vi "SubVI_Overlay Result.vi"(8 "Error in":errorcluster, 9 "Parameter_String":T1={"Font, Size & Style"={"Desired Font (Application)"=enum."Application Font", "[User-specified Font]"={"Font Name"="", "Size"=12, "Strikeout?"=FALSE, "Italic?"=FALSE, "Underline?"=FALSE, "Outline?"=FALSE, "Shadow?"=FALSE, "Bold?"=FALSE, "Rotation Angle"=0.0}, "Horizontal Alignment"=0, "Vertical Alignment"=0}, "Position"={"Image X %"=5.0, "Image Y %"=5.0}} {"Position"."Image Y %" min=5 max=95 step=5; "Position"."Image X %" min=5 max=95 step=5; "Font, Size & Style"."Vertical Alignment" items=["Bottom", "Top", "Baseline"]; "Font, Size & Style"."Horizontal Alignment" items=["Left", "Center", "Right"]; "Font, Size & Style"."[User-specified Font]"."Rotation Angle" format="%.2f"}, 10 "Result Array":T3(array[cluster]), 11 "Image In":T2) -> ()   [LabVIEW 2013]
uses:
  <vilib>/vision/Image Controls.llb/IMAQ Image.ctl
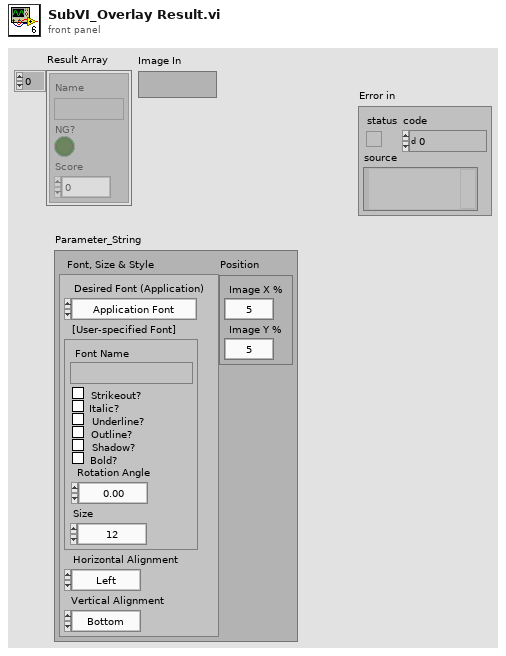
[diagram p1: front panel]
types:
  T1 = cluster{"Font, Size & Style":cluster{"Desired Font (Application)":enum16{"User-specified Font", "Application Font", "System Font", "Dialog Font"}, "[User-specified Font]":cluster{"Font Name":string, "Size":i16, "Strikeout?":bool, "Italic?":bool, "Underline?":bool, "Outline?":bool, "Shadow?":bool, "Bold?":bool, "Rotation Angle":dbl}, "Horizontal Alignment":i16, "Vertical Alignment":i16}, "Position":cluster{"Image X %":sgl, "Image Y %":sgl}}
  T2 = typedef "IMAQ Image.ctl" = refnum<image>
  T3 = cluster{"Name":string, "NG?":bool, "Score":dbl}[]
  T4 = cluster{"Desired Font (Application)":enum16{"User-specified Font", "Application Font", "System Font", "Dialog Font"}, "[User-specified Font]":cluster{"Font Name":string, "Size":i16, "Strikeout?":bool, "Italic?":bool, "Underline?":bool, "Outline?":bool, "Shadow?":bool, "Bold?":bool, "Rotation Angle":dbl}, "Horizontal Alignment":i16, "Vertical Alignment":i16}
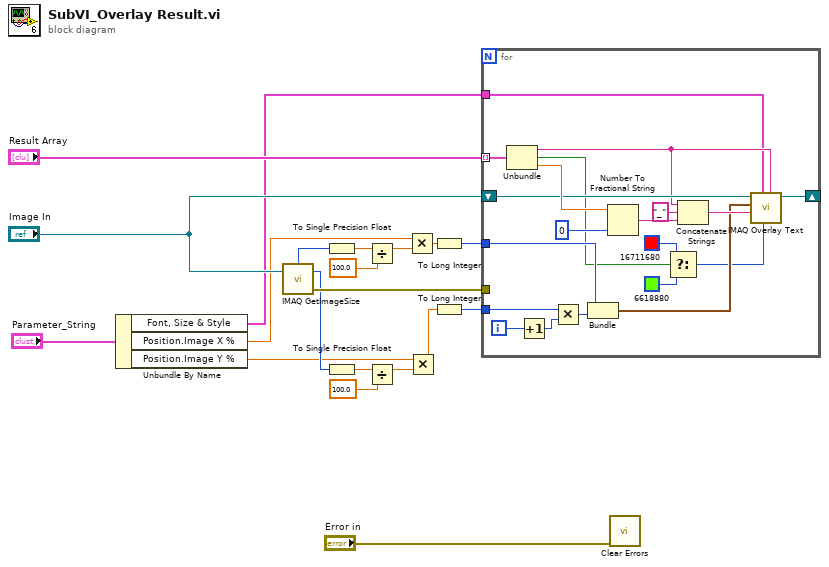
[diagram p0: block diagram]
diagram:
  n1 = Unbundle By Name("Parameter_String") -> ("Font, Size & Style"=w7:T4, "Position.Image X %"=w8:sgl, "Position.Image Y %"=w9:sgl)
  n2 = call "IMAQ GetImageSize"("Image"="Image In") -> ("Y Resolution"=w13:i32, "X Resolution"=w18:i32, "error out"=w20:errorcluster)  [unwired: 3 in]
  n3 = To Single Precision Float(number=w18) -> (single precision float=w6:sgl)
  n4 = To Single Precision Float(number=w13) -> (single precision float=w2:sgl)
  n5 = Divide(x=w6, y=sgl 100.0) -> (x/y=w5:sgl)
  n6 = Divide(x=w2, y=sgl 100.0) -> (x/y=w1:sgl)
  n7 = Multiply(x=w8, y=w5) -> (x*y=w17:sgl)
  n8 = Multiply(x=w9, y=w1) -> (x*y=w11:sgl)
  n9 = To Long Integer(number=w17) -> (32bit integer=w16:i32)
  n10 = To Long Integer(number=w11) -> (32bit integer=w12:i32)
  n11 = for {
    tunnel: "Result Array" -> [w40] mode=indexing
    tunnel: w7 -> [w21]
    tunnel: w20 -> [_]
    tunnel: w16 -> [w33]
    tunnel: w12 -> [w34]
    shift-right: [w27] -> _
    shift-left: "Image In" -> [w35]
    i -> [w24]
    n12 = Unbundle(w40) -> ("Name"=w26:string, "NG?"=w30:bool, "Score"=w38:dbl)
    n13 = Increment(x=w24) -> (x+1=w23:i32)
    n14 = Multiply(x=w34, y=w23) -> (x*y=w32:i32)
    n15 = Bundle(w33, w32) -> (w31:cluster{i32, i32})  [unwired: 1 in]
    n16 = Number To Fractional String(number=w38, precision (6)=i16 0) -> (F-format string=w37:string)  [unwired: 2 in]
    n17 = Select(t=u32 16711680 ("Text Color (black)"), s=w30, f=u32 6618880 ("Text Color (black)")) -> (s? t:f=w22:u32)
    n18 = Concatenate Strings(w26, "_" ("string"), w37) -> (w39:string)
    n19 = call "IMAQ Overlay Text"("Group"=w26, "Text Color (black)"=w22, "Font, Size & Style"=w21, "String"=w39, "Origin"=w31, "Image"=w35) -> ("Image Out"=w27:T2)  [unwired: 4 in, 1 out]
  }
  n20 = call <vilib>:"Clear Errors.vi"("error in (no error)"="Error in") -> ()  [unwired: 6 in, 1 out]
